vi "FRCts20_WebMethods_ESP_CommentForm.vi"(8 "error in (no error)":errorcluster, 10 "Return Type":T1="mobile", 11 "httpRequestID":u32) -> (0 "error out":errorcluster, 3 "httpRequestID out":u32)   [LabVIEW 2014]
uses:
  Controls/FRCts20_WebMethods_ctl_returntype.ctl
  Controls/FRCts20_WebMethods_Globals.vi
  <vilib>/wsapi/subVIs/Set String ESP Variable.vi
  <vilib>/wsapi/subVIs/Set Integer ESP Variable.vi
  <vilib>/wsapi/NI_WebServices.lvlib
  FRCts20_WebMethods.lvlib
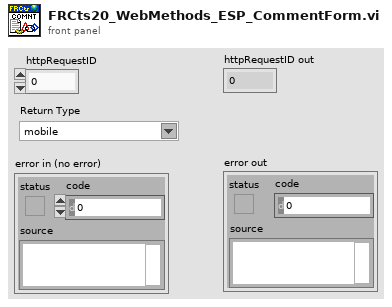
[diagram p1: front panel]
types:
  T1 = typedef "FRCts20_WebMethods.lvlib/FRCts20_WebMethods_ctl_returntype.ctl" = string
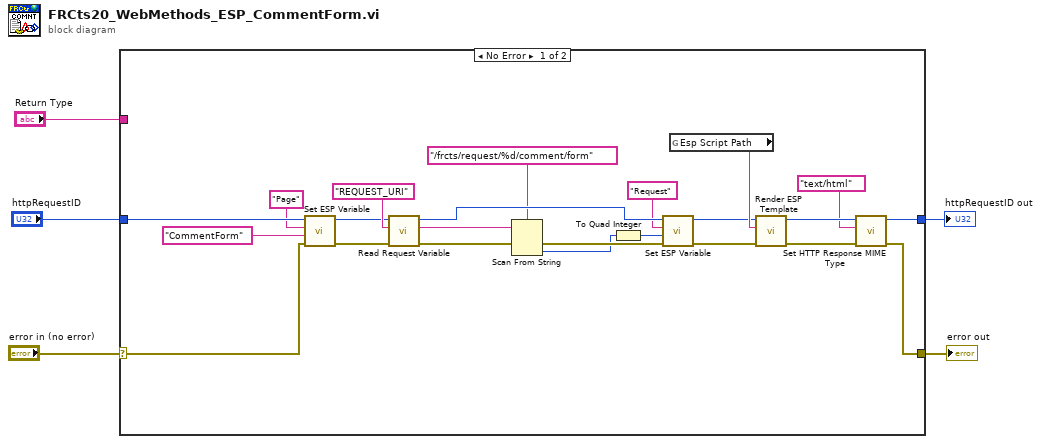
[diagram p0: block diagram]
diagram:
  n1 = case shown="No Error" "error in (no error)" {
    selector: "error in (no error)" -> [w16 w30]
    tunnel: "httpRequestID" -> [w22 w29]
    tunnel: [w26 w29] -> w2
    tunnel: [w25 w30] -> w1
    tunnel: "Return Type" -> [_ _]
    frame No Error {
      n2 = call-poly <vilib>:"Set ESP Variable.vi"("error in (no error)"=w16, "value"="CommentForm", "key"="Page", "httpRequestID"=w22) -> ("error out"=w17:errorcluster, "httpRequestID out"=w18:u32)  [unwired: 6 in]
      n3 = call <vilib>:"Read Request Variable.vi"("error in (no error)"=w17, "variable name"="REQUEST_URI", "httpRequestID"=w18) -> ("error out"=w14:errorcluster, "value"=w15:string, "httpRequestID out"=w12:u32)  [unwired: 6 in]
      n4 = Scan From String(format string="/frcts/request/%d/comment/form", input string=w15, error in=w14) -> (error out=w13:errorcluster, output 1=w6:i32)  [unwired: 2 in, 2 out]
      n5 = To Quad Integer(1:w6) -> (0:w7:i64)
      n6 = call-poly <vilib>:"Set ESP Variable.vi"("error in (no error)"=w13, "value"=w7, "key"="Request", "httpRequestID"=w12) -> ("error out"=w9:errorcluster, "httpRequestID out"=w10:u32)  [unwired: 6 in]
      n7 = global read "FRCts20_WebMethods_Globals.vi" "Esp Script Path"() -> (w24:string)
      n8 = call <vilib>:"Render ESP Template.vi"("error in (no error)"=w9, "espName"=w24, "httpRequestID"=w10) -> ("error out"=w27:errorcluster, "httpRequestID out"=w28:u32)  [unwired: 7 in]
      n9 = call <vilib>:"Set HTTP Response MIME Type.vi"("error in (no error)"=w27, "MIME type (text/html)"="text/html", "httpRequestID"=w28) -> ("error out"=w25:errorcluster, "httpRequestID out"=w26:u32)  [unwired: 7 in]
    }
    frame Error {
    }
  }
  "httpRequestID out" <- w2
  "error out" <- w1
